vi "getAhmedTaps.vi"() -> (1 "MAP":string[][](array[string]), 2 "Y":dbl[][](array[numeric]), 3 "X":dbl[][](array[numeric]))   [LabVIEW 2017]
uses:
  <vilib>/Utility/file.llb/Read Delimited Spreadsheet (DBL).vi
  <vilib>/Utility/file.llb/Read Delimited Spreadsheet (string).vi
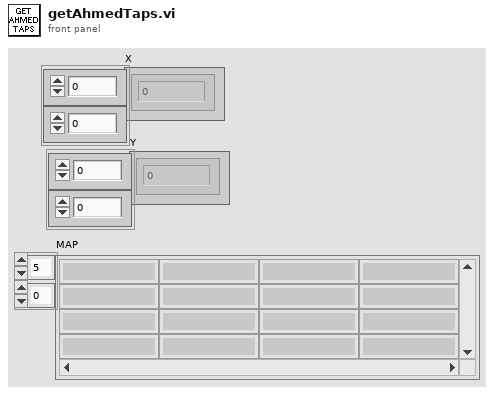
[diagram p1: front panel]
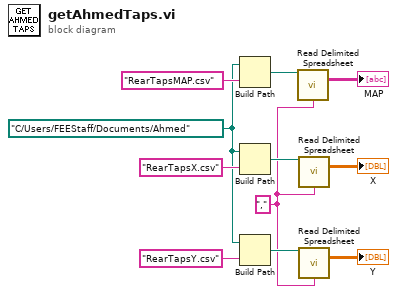
[diagram p0: block diagram]
diagram:
  w2 = "," ("delimiter (\\t)")
  w4 = path "C:/Users/FEEStaff/Documents/Ahmed" ("File Path Control")
  n1 = Build Path(base path=w4, name or relative path="RearTapsMAP.csv") -> (appended path=w3:path)
  n2 = Build Path(base path=w4, name or relative path="RearTapsX.csv") -> (appended path=w8:path)
  n3 = Build Path(base path=w4, name or relative path="RearTapsY.csv") -> (appended path=w10:path)
  n4 = call-poly <vilib>:"Read Delimited Spreadsheet.vi"("file path (dialog if empty)"=w3, "delimiter (\\t)"=w2) -> ("all rows"=→"MAP":string[][])  [unwired: 8 in, 5 out]
  n5 = call-poly <vilib>:"Read Delimited Spreadsheet.vi"("file path (dialog if empty)"=w8, "delimiter (\\t)"=w2) -> ("all rows"=→"X":dbl[][])  [unwired: 8 in, 5 out]
  n6 = call-poly <vilib>:"Read Delimited Spreadsheet.vi"("file path (dialog if empty)"=w10, "delimiter (\\t)"=w2) -> ("all rows"=→"Y":dbl[][])  [unwired: 8 in, 5 out]
